vi "Untitled 1.vi"() -> ()   [LabVIEW 2019]
panel:
  in  "RESET 2":bool
  in  "Tab Control":enum32{"Motor 1", "Motor 2"}(tab)
  out "Waveform Chart 6":waveform(dbl)[](graph)
  out "Waveform Chart 5":waveform(dbl)[](graph)
  out "Hall 1":bool
  out "Posición":waveform(dbl)[](graph)
  out "Hall 3":bool
  out "Waveform Chart 4":waveform(dbl)[](graph)
  out "Waveform Chart 3":waveform(dbl)[](graph)
  out "Hall 2":bool
  out "Waveform Chart 2":waveform(dbl)[](graph)
  out "Hall1":bool
  in  "Home":bool
  in  "GO 2":bool
  in  "RESET 1":bool
  in  "GO":bool
  in  "Stop UI and RT":bool
  in  "Stop UI":bool
  in  "Posición final Motor 2":dbl caption="Posición final motor 2"
  in  "Velocidad inicial Motor 2":dbl
  in  "Velocidad final Motor 2":dbl
  in  "Aceleración inicial Motor 2":dbl
  in  "Aceleración final Motor 2":dbl
  in  "Tiempo 2":dbl
  in  "Posición final motor 1":dbl caption="Posición final en X"
  in  "Velocidad inicial Motor 1":dbl caption="Posición final en Y"
  in  "Velocidad final Motor 1":dbl
  in  "Aceleración inicial Motor 1":dbl
  in  "Aceleración final Motor 1":dbl
  in  "Tiempo 1":dbl
  in  "Trayectoria:":bool
  out "String":string
  in  "Motores independientes":bool
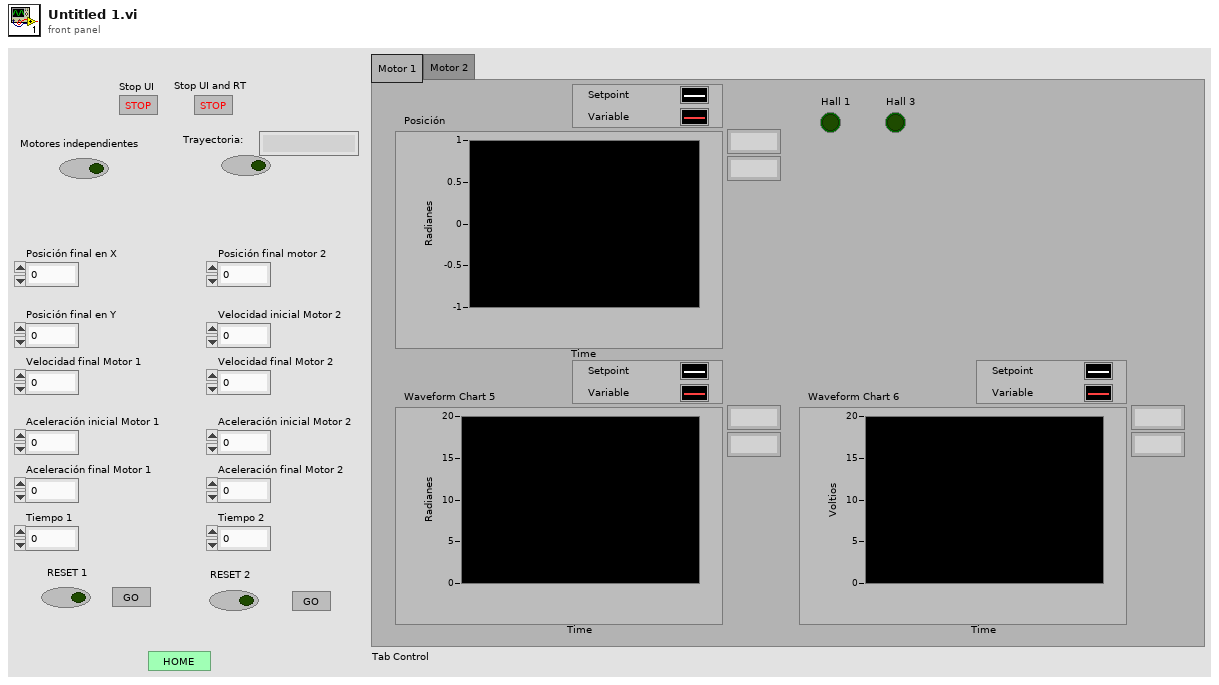
[diagram p1: front panel]
types:
  T1 = cluster{"Double":dbl, "dbl Scaled Value":dbl, "Output":dbl, "seconds since 1Jan1904":timestamp}
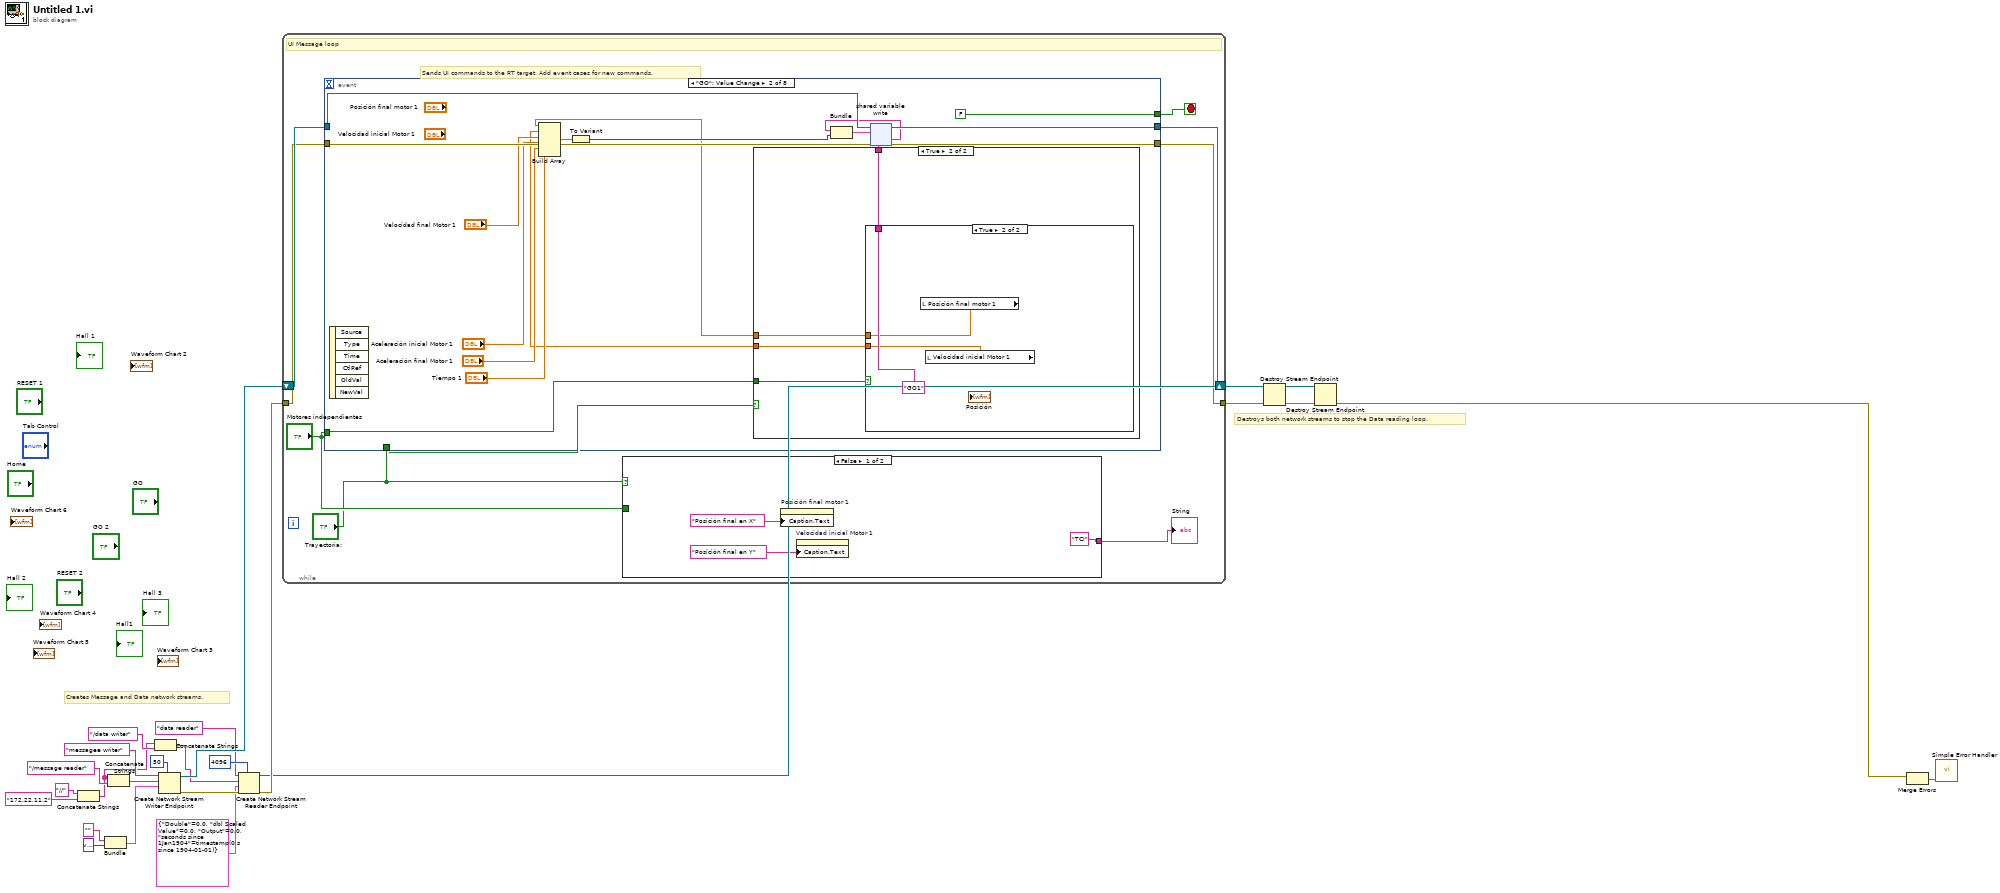
[diagram p0: block diagram]
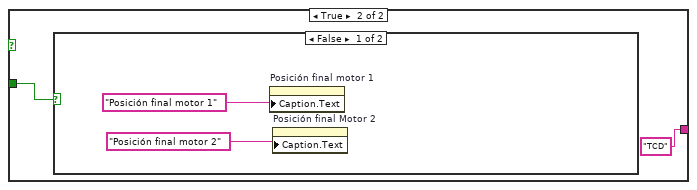
[diagram p2: hidden frame]
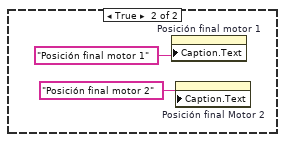
[diagram p3: hidden frame]
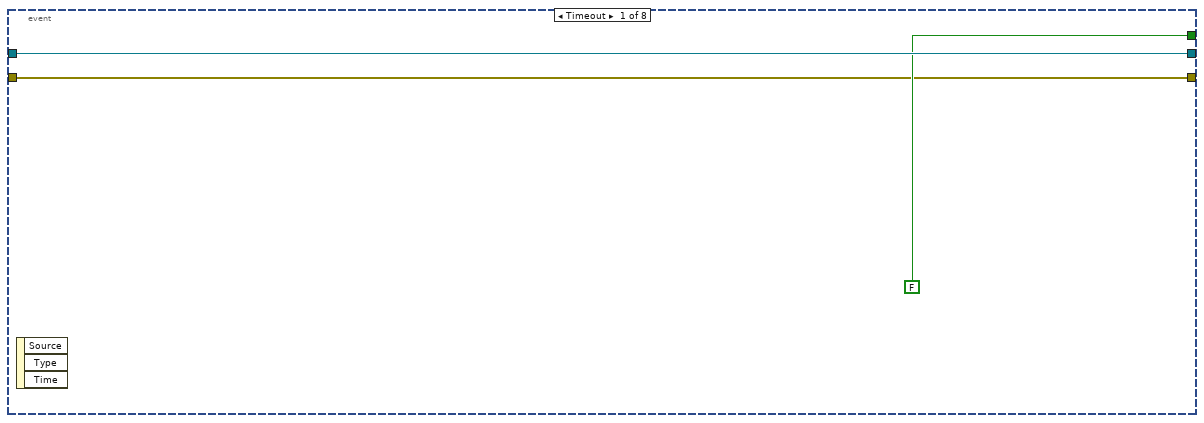
[diagram p4: hidden frame]
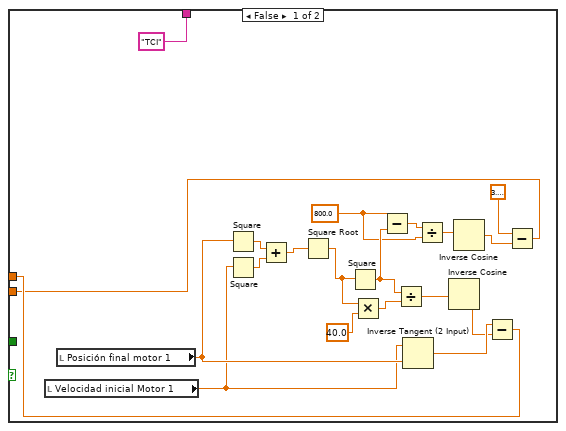
[diagram p5: hidden frame]
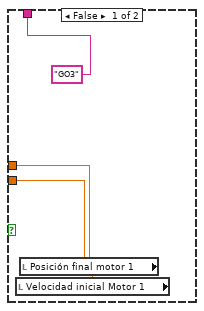
[diagram p6: hidden frame]
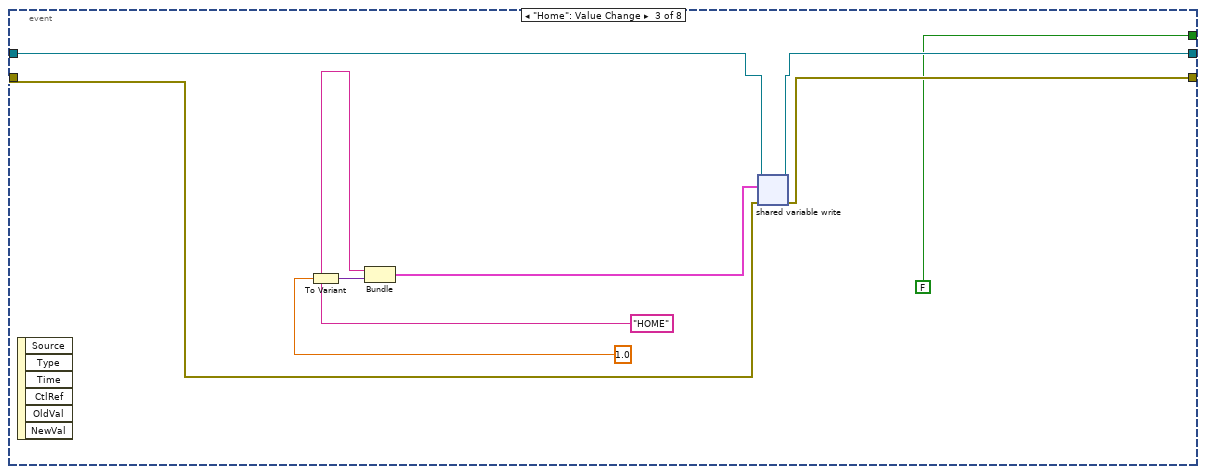
[diagram p7: hidden frame]
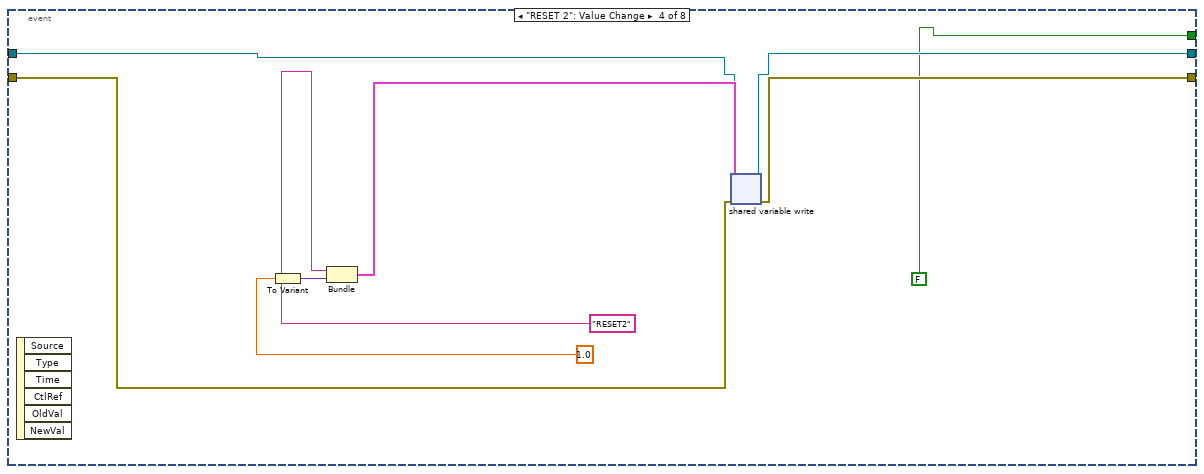
[diagram p8: hidden frame]
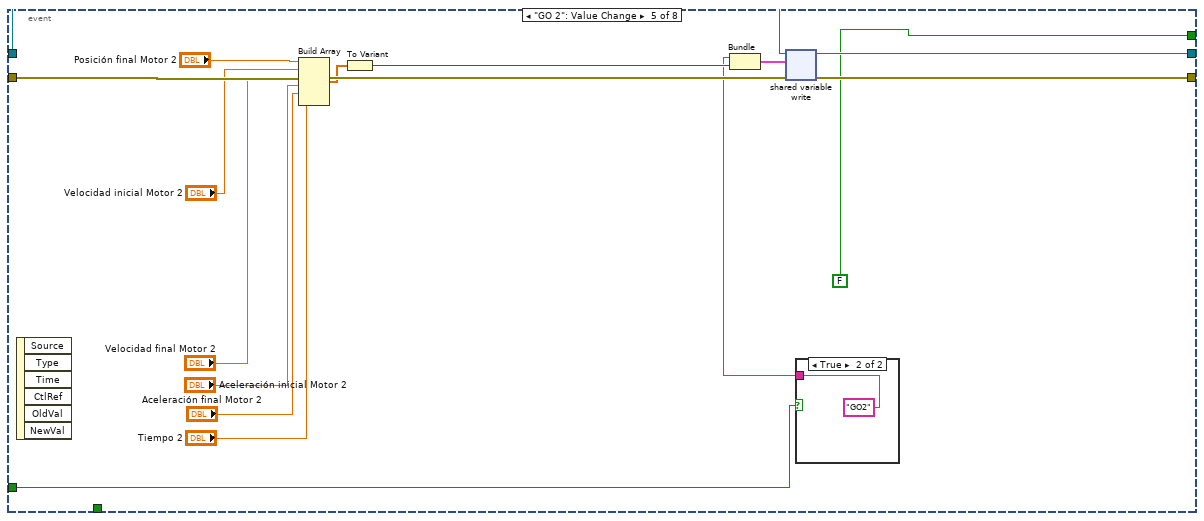
[diagram p9: hidden frame]
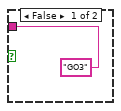
[diagram p10: hidden frame]
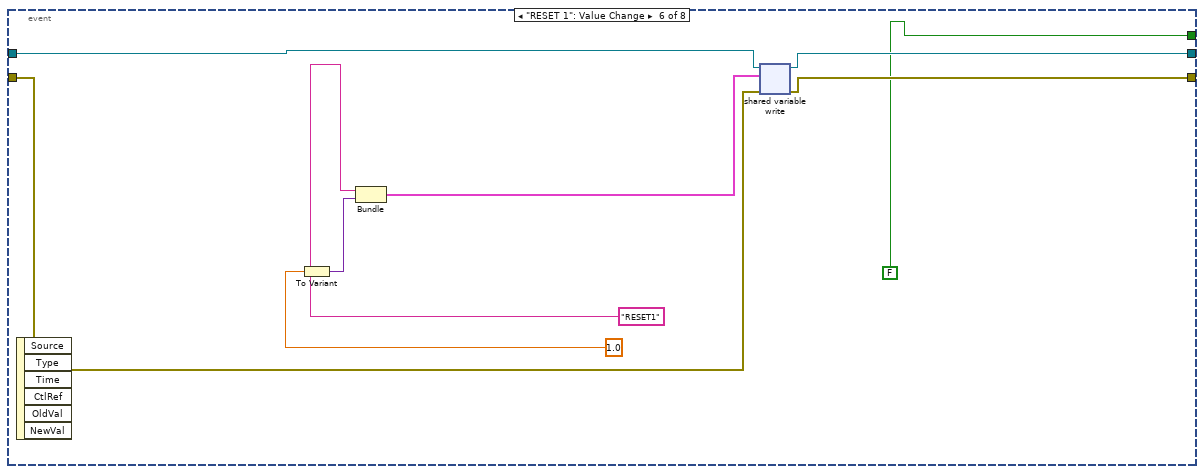
[diagram p11: hidden frame]
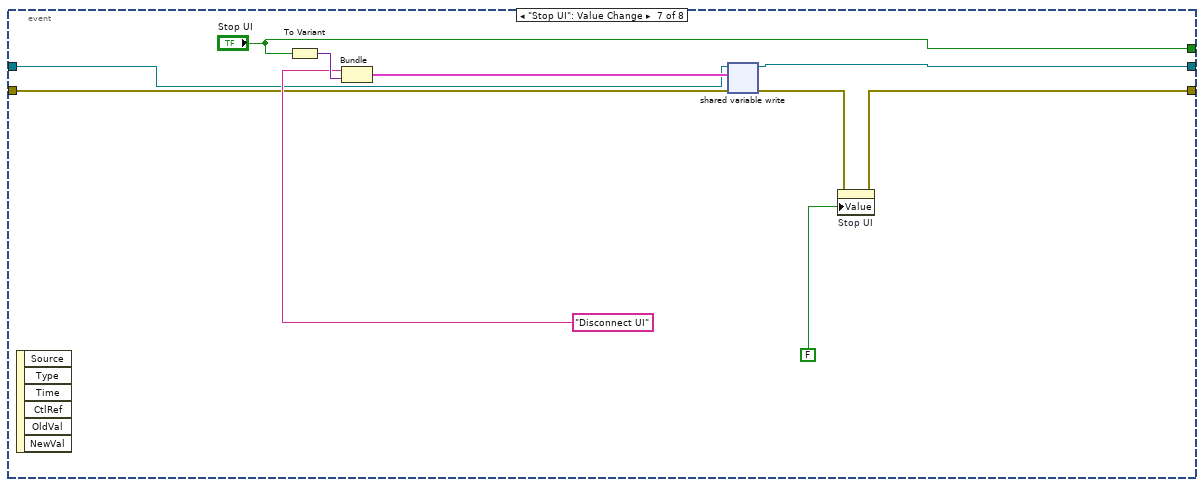
[diagram p12: hidden frame]
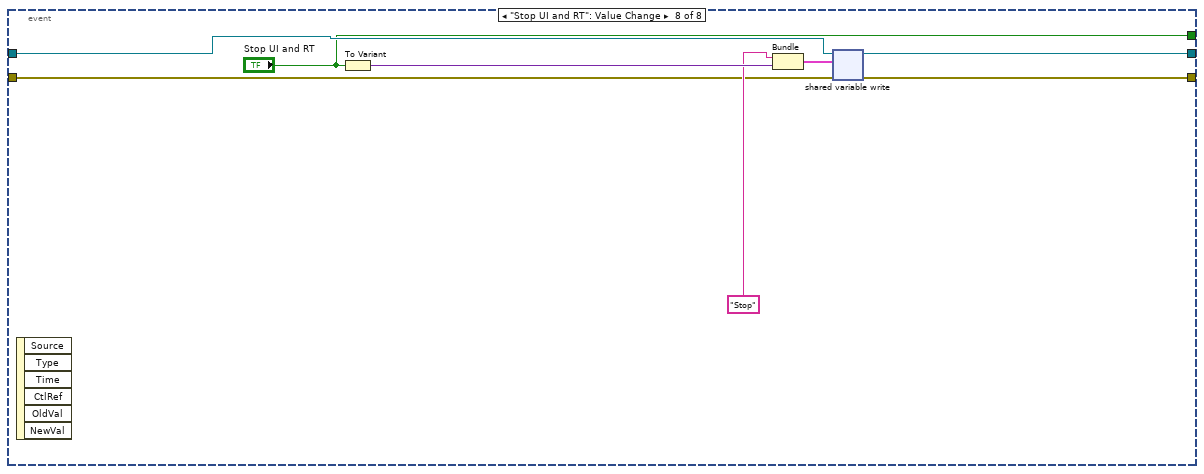
[diagram p13: hidden frame]
diagram:
  # "Destroys both network streams to stop the Data reading loop."
  # "Creates Message and Data network streams."
  n1 = Concatenate Strings("//", "172.22.11.2" ("myRIO IP")) -> (w1:string)
  n2 = Bundle("", variant) -> (w25:cluster{string, variant})  [unwired: 1 in]
  n3 = Concatenate Strings(w1, "/message reader") -> (w2:string)
  n4 = Concatenate Strings(w1, "/data writer") -> (w16:string)
  n5 = Create Network Stream Writer Endpoint(7:50 ("writer buffer size"), 9:w25, 10:w2, 11:"messagee writer" ("writer name")) -> (0:w13:errorcluster, 3:w19:refnum<k21>)  [unwired: 3 in]
  n6 = Create Network Stream Reader Endpoint(7:4096 ("reader buffer size"), 8:w13, 9:T1 {"Double"=0.0, "dbl Scaled Value"=0.0, "Output"=0.0, "seconds since 1Jan1904"=timestamp(0 s since 1904-01-01)} ("Data"), 10:w16, 11:"data reader" ("reader name")) -> (0:w12:errorcluster, 3:w5:refnum<k21>)  [unwired: 2 in]
  n7 = while {
    tunnel: w12 -> [w32]
    shift-right: [w31] -> w7
    shift-left: w19 -> [w33]
    tunnel: [w30] -> w8
    stop <- w29 stop-if-true
    # "Sends UI commands to the RT target. Add event cases for new commands."
    # "UI Message loop"
    n8 = event shown="[1] \"GO\": Value Change" {
      selector: _ -> [_ _ _ _ _ _ _ _]
      dyn-events: _ -> [_ _ _ _ _ _ _ _]
      timeout: _ -> [_ _ _ _ _ _ _ _]
      tunnel: w33 -> [w45 w62 w98 w104 w123 w132 w144 w149]
      tunnel: w32 -> [w43 w61 w95 w103 w121 w130 w140 w152]
      tunnel: [w45 w58 w97 w105 w124 w133 w143 w150] -> w31
      tunnel: [w43 w57 w96 w106 w122 w131 w138 w151] -> w30
      tunnel: [FALSE ("Stop UI and RT") FALSE ("Stop UI and RT") FALSE FALSE ("Stop UI and RT") FALSE ("Stop UI and RT") FALSE ("Stop UI and RT") "Stop UI" "Stop UI and RT"] -> w29
      tunnel: "Motores independientes" -> [_ w52 _ _ w113 _ _ _]
      tunnel: "Trayectoria:" -> [_ w48 _ _ _ _ _ _]
      event Timeout {
        n9 = event-data() -> ()  [unwired: 1 in, 3 out]
      }
      event "GO": Value Change {
        n10 = event-data() -> ()  [unwired: 1 in, 6 out]
        n11 = case shown="True" w48 {
          tunnel: ["TCI" w86] -> w55
          tunnel: w52 -> [_ w85]
          tunnel: [w66 w84] -> w47
          tunnel: [w63 w83] -> w46
          frame False {
            w71 = 800.0
            n12 = local read "Velocidad inicial Motor 1"() -> (w69:dbl)
            n13 = local read "Posición final motor 1"() -> (w70:dbl)
            n14 = Square(x=w70) -> (x^2=w81:dbl)
            n15 = Square(x=w69) -> (x^2=w80:dbl)
            n16 = Add(x=w81, y=w80) -> (x+y=w79:dbl)
            n17 = Square Root(x=w79) -> (sqrt(x)=w75:dbl)
            n18 = Square(x=w75) -> (x^2=w74:dbl)
            n19 = Multiply(x=w75, y=40.0) -> (x*y=w76:dbl)
            n20 = Subtract(x=w71, y=w74) -> (x-y=w72:dbl)
            n21 = Divide(x=w74, y=w76) -> (x/y=w78:dbl)
            n22 = Inverse Tangent (2 Input)(1:w70, 2:w69) -> (0:w68:dbl)
            n23 = Divide(x=w72, y=w71) -> (x/y=w73:dbl)
            n24 = Inverse Cosine(1:w78) -> (0:w67:dbl)
            n25 = Inverse Cosine(1:w73) -> (0:w64:dbl)
            n26 = Subtract(x=w68, y=w67) -> (x-y=w66:dbl)
            n27 = Subtract(x=3.141592653589793, y=w64) -> (x-y=w63:dbl)
          }
          frame True {
            n28 = case shown="True" w85 {
              tunnel: ["GO3" ("writer name") "GO1" ("writer name")] -> w86
              tunnel: [w88 w90] -> w84
              tunnel: [w87 w91] -> w83
              frame False {
                n29 = local read "Velocidad inicial Motor 1"() -> (w87:dbl)
                n30 = local read "Posición final motor 1"() -> (w88:dbl)
              }
              frame True {
                n31 = local read "Posición final motor 1"() -> (w90:dbl)
                n32 = local read "Velocidad inicial Motor 1"() -> (w91:dbl)
              }
            }
          }
        }
        n33 = Build Array(w47, w46, "Velocidad final Motor 1", "Aceleración inicial Motor 1", "Aceleración final Motor 1", "Tiempo 1") -> (w54:dbl[])
        n34 = To Variant(anything=w54) -> (Variant=w60:variant)
        n35 = Bundle("writer name"=w55, "Variant"=w60) -> (w59:cluster{"writer name":string, "Variant":variant})  [unwired: 1 in]
        n36 = shared-variable-write(w62, w61, w59) -> (w58:refnum<k21>, w57:errorcluster)  [unwired: 1 in, 1 out]
      }
      event "Home": Value Change {
        n37 = event-data() -> ()  [unwired: 1 in, 6 out]
        n38 = To Variant(anything=1.0) -> (Variant=w101:variant)
        n39 = Bundle("writer name"="HOME", "Variant"=w101) -> (w99:cluster{"writer name":string, "Variant":variant})  [unwired: 1 in]
        n40 = shared-variable-write(w98, w95, w99) -> (w97:refnum<k21>, w96:errorcluster)  [unwired: 1 in, 1 out]
      }
      event "RESET 2": Value Change {
        n41 = event-data() -> ()  [unwired: 1 in, 6 out]
        n42 = To Variant(anything=1.0) -> (Variant=w109:variant)
        n43 = Bundle("writer name"="RESET2", "Variant"=w109) -> (w110:cluster{"writer name":string, "Variant":variant})  [unwired: 1 in]
        n44 = shared-variable-write(w104, w103, w110) -> (w105:refnum<k21>, w106:errorcluster)  [unwired: 1 in, 1 out]
      }
      event "GO 2": Value Change {
        n45 = event-data() -> ()  [unwired: 1 in, 6 out]
        n46 = Build Array("Posición final Motor 2", "Velocidad inicial Motor 2", "Velocidad final Motor 2", "Aceleración inicial Motor 2", "Aceleración final Motor 2", "Tiempo 2") -> (w119:dbl[])
        n47 = To Variant(anything=w119) -> (Variant=w126:variant)
        n48 = case shown="True" w113 {
          tunnel: ["GO3" ("writer name") "GO2" ("writer name")] -> w112
          frame False {
          }
          frame True {
          }
        }
        n49 = Bundle("writer name"=w112, "Variant"=w126) -> (w125:cluster{"writer name":string, "Variant":variant})  [unwired: 1 in]
        n50 = shared-variable-write(w123, w121, w125) -> (w124:refnum<k21>, w122:errorcluster)  [unwired: 1 in, 1 out]
      }
      event "RESET 1": Value Change {
        n51 = event-data() -> ()  [unwired: 1 in, 6 out]
        n52 = To Variant(anything=1.0) -> (Variant=w136:variant)
        n53 = Bundle("writer name"="RESET1", "Variant"=w136) -> (w137:cluster{"writer name":string, "Variant":variant})  [unwired: 1 in]
        n54 = shared-variable-write(w132, w130, w137) -> (w133:refnum<k21>, w131:errorcluster)  [unwired: 1 in, 1 out]
      }
      event "Stop UI": Value Change {
        n55 = event-data() -> ()  [unwired: 1 in, 6 out]
        n56 = To Variant(anything="Stop UI") -> (Variant=w147:variant)
        n57 = Bundle("writer name"="Disconnect UI", "Variant"=w147) -> (w146:cluster{"writer name":string, "Variant":variant})  [unwired: 1 in]
        n58 = shared-variable-write(w144, w140, w146) -> (w143:refnum<k21>, w139:errorcluster)  [unwired: 1 in, 1 out]
        n59 = property on="Stop UI" class="Bool (strict)"(error in=w139, "Value"=FALSE ("Stop UI and RT")) -> (error out=w138:errorcluster)  [unwired: 1 in, 1 out]
      }
      event "Stop UI and RT": Value Change {
        n60 = event-data() -> ()  [unwired: 1 in, 6 out]
        n61 = To Variant(anything="Stop UI and RT") -> (Variant=w155:variant)
        n62 = Bundle("writer name"="Stop", "Variant"=w155) -> (w154:cluster{"writer name":string, "Variant":variant})  [unwired: 1 in]
        n63 = shared-variable-write(w149, w152, w154) -> (w150:refnum<k21>, w151:errorcluster)  [unwired: 1 in, 1 out]
      }
    }
    n64 = case shown="False" "Trayectoria:" {
      tunnel: ["TCI" "TCD"] -> w28
      tunnel: "Motores independientes" -> [_ w37]
      frame False {
        n65 = property on="Posición final motor 1" class="DigNum (strict)"("Caption.Text"="Posición final en X") -> ()  [unwired: 2 in, 2 out]
        n66 = property on="Velocidad inicial Motor 1" class="DigNum (strict)"("Caption.Text"="Posición final en Y") -> ()  [unwired: 2 in, 2 out]
      }
      frame True {
        n67 = case shown="False" w37 {
          frame False {
            n68 = property on="Posición final motor 1" class="DigNum (strict)"("Caption.Text"="Posición final motor 1") -> ()  [unwired: 2 in, 2 out]
            n69 = property on="Posición final Motor 2" class="DigNum (strict)"("Caption.Text"="Posición final motor 2") -> ()  [unwired: 2 in, 2 out]
          }
          frame True {
            n70 = property on="Posición final motor 1" class="DigNum (strict)"("Caption.Text"="Posición final motor 1") -> ()  [unwired: 2 in, 2 out]
            n71 = property on="Posición final Motor 2" class="DigNum (strict)"("Caption.Text"="Posición final motor 2") -> ()  [unwired: 2 in, 2 out]
          }
        }
      }
    }
    "String" <- w28
  }
  n72 = Destroy Stream Endpoint(8:w8, 11:w7) -> (0:w6:errorcluster)
  n73 = Destroy Stream Endpoint(8:w6, 11:w5) -> (0:w4:errorcluster)
  n74 = Merge Errors(w4) -> (w10:errorcluster, w9:errorcluster)
  n75 = call <vilib>:"Simple Error Handler.vi"("error in (no error)"=w10) -> ()  [unwired: 4 in, 5 out]
